vi "SerialTest.vi"() -> ()   [LabVIEW 2012]
panel:
  in  "Send":bool
  in  "string 2":string
  in  "stop":bool
  out "string":string
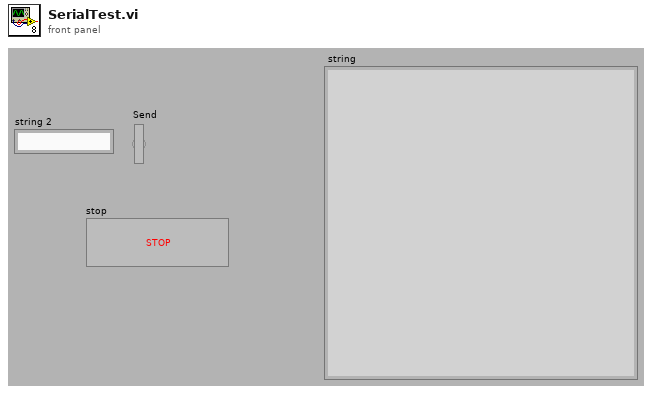
[diagram p1: front panel]
types:
  T1 = typedef "URAPI_Control.ctl" = cluster{"Script":string, "Whiles":u8[], "Ifs":u8[], "remote":bool, "RIO Settings":T2, "Supress Err":bool}
  T2 = typedef "RIO_Control.ctl" = cluster{"IP Address":string, "Connected?":bool, "connection ID":refnum<k5>, "Script":string}
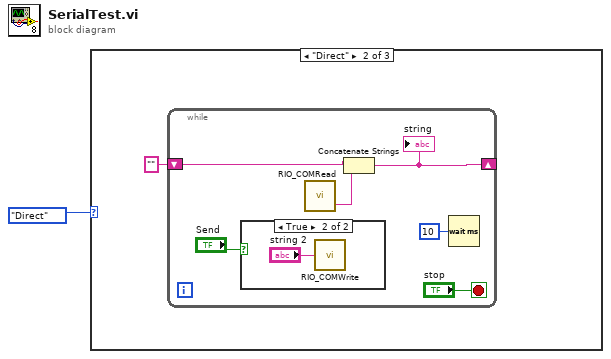
[diagram p0: block diagram]
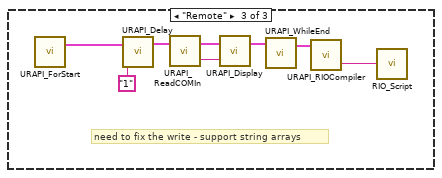
[diagram p4: hidden frame]
diagram:
  n1 = case shown="\"Direct\"" enum16{"Direct", "Remote"}."Direct" {
    frame Default {
    }
    frame "Direct" {
      n2 = while {
        shift-right: [w7] -> _
        shift-left: "" -> [w6]
        stop <- "stop" stop-if-true
        n3 = case shown="True" "Send" {
          frame False {
          }
          frame True {
            n4 = call <userlib>:"RIO_COMWrite.vi"("string"="string 2") -> ()  [unwired: 3 in, 1 out]
          }
        }
        n5 = call <userlib>:"RIO_COMRead.vi"() -> ("response"=w8:string)  [unwired: 3 in, 1 out]
        n6 = Concatenate Strings(w6, w8) -> (w7:string)
        "string" <- w7
        n7 = Wait (ms)(milliseconds to wait=u32 10) -> ()  [unwired: 1 out]
      }
    }
    frame "Remote" {
      # "need to fix the write - support string arrays"
      n8 = call <userlib>:"URAPI_ForStart.vi"() -> ("URAPI Script Out"=w10:T1)  [unwired: 4 in, 1 out]
      n9 = call <userlib>:"URAPI_Delay.vi"("Variable In"="1", "URAPI Script"=w10) -> ("URAPI Script out"=w13:T1)  [unwired: 3 in]
      n10 = call <userlib>:"URAPI_ReadCOMIn.vi"("URAPI Script"=w13) -> ("Variable Out"=w17:string, "URAPI Script"=w16:T1)  [unwired: 3 in]
      n11 = call <userlib>:"URAPI_Display.vi"("Variable In"=w17, "URAPI Script"=w16) -> ("URAPI Script"=w15:T1)  [unwired: 2 in, 1 out]
      n12 = call <userlib>:"URAPI_WhileEnd.vi"("URAPI Script"=w15) -> ("URAPI Script Out"=w14:T1)  [unwired: 4 in]
      n13 = call <userlib>:"URAPI_RIOCompiler.vi"("URAPI Script"=w14) -> ("Script"=w11:string)  [unwired: 4 in]
      n14 = call <userlib>:"RIO_Script.vi"("Script"=w11) -> ()  [unwired: 3 in, 1 out]
    }
  }
